vi "Initialize.vi"(8 "error in (no error)":errorcluster, 9 "Protocol Type":T1, 10 "Folder Path":path, 11 "Protocol Interface in":refnum<class "Protocol Interface.lvclass">) -> (0 "error out":errorcluster, 3 "Protocol Interface out":refnum<class "Protocol Interface.lvclass">)   [LabVIEW 2018, in "Protocol Interface.lvlib" / "Protocol Interface.lvclass"]
uses:
  Protocol Interface.lvclass
  Ctls/Protocol Type.ctl
  Protocol Interface.lvclass/Protocol Interface.ctl
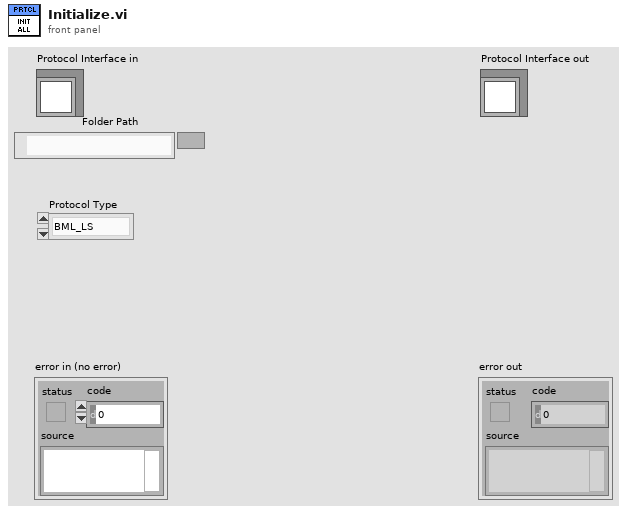
[diagram p1: front panel]
types:
  T1 = typedef "Protocol Type.ctl" = enum16{"BML_LS", "BML_HS", "SPI_3W", "SPI_4W"}
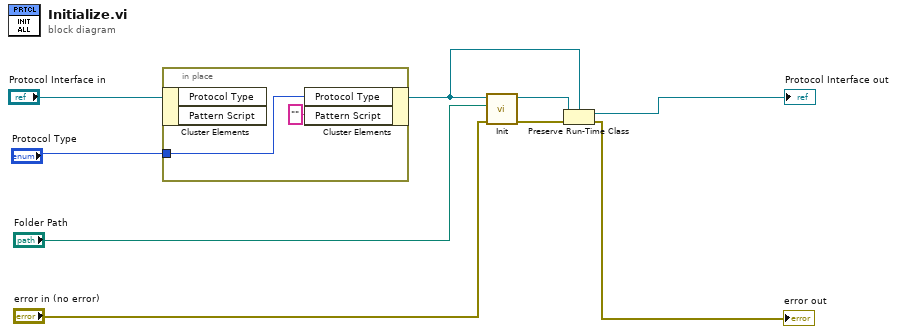
[diagram p0: block diagram]
diagram:
  n1 = in-place {
    in-place-border: "Protocol Type" -> [w11]
    n2 = in-place-cluster #1("Protocol Interface in") -> ()  [unwired: 2 out]
    n3 = in-place-cluster #1("Protocol Type"=w11, "Pattern Script"="") -> (w4:refnum<class "Protocol Interface.lvclass">)
  }
  n4 = call-dynamic "Init.vi"("Error In"="error in (no error)", "Folder Path"="Folder Path", "Protocol Interface in"=w4) -> ("Error Out"=w3:errorcluster, "Protocol Interface out"=w5:refnum<class "Protocol Interface.lvclass">)  [unwired: 7 in]
  n5 = Preserve Run-Time Class(object in=w5, error in=w3, 2:w4) -> (object out=→"Protocol Interface out":refnum<class "Protocol Interface.lvclass">, error out=→"error out":errorcluster)
